vi "Three Sensors.vi"() -> ()   [LabVIEW 2019]
uses:
  <vilib>/Platform/TimedLoop/XDataNode/timing_clust.ctl
  <vilib>/Platform/TimedLoop/XDataNode/nitl_modes.ctl
  <vilib>/Platform/TimedLoop/XDataNode/wakeup.ctl
  <vilib>/myRIO/Instrument Drivers/Onboard IO/I2C/typedefs/I2C User Configuration.ctl
  <vilib>/myRIO/Instrument Drivers/Onboard IO/I2C/typedefs/I2C Transfer Rate.ctl
  <vilib>/myRIO/Instrument Drivers/Onboard IO/I2C/typedefs/I2C Reference.ctl
  <vilib>/myRIO/Common/Instrument Driver Framework/Utilities/typedefs/myRIO Generic Hardware Reference.ctl
  <vilib>/myRIO/Common/Instrument Driver Framework/Utilities/typedefs/Hardware Version Enum.ctl
  <vilib>/myRIO/Common/Instrument Driver Framework/Utilities/typedefs/myRIO v1.0 Reference.ctl
  <vilib>/myRIO/Common/Instrument Driver Framework/Utilities/typedefs/Generic FPGA Reference.ctl
  <vilib>/myRIO/Common/Instrument Driver Framework/myRIO v1.0/I2C/typedefs/I2C Channels Enum.ctl
  <vilib>/myRIO/Instrument Drivers/Onboard IO/I2C/typedefs/I2C Configuration.ctl
  <vilib>/userDefined/High Color/nirio_resource_hc.ctl
  <vilib>/myRIO/Common/Instrument Driver Framework/Utilities/vis/Is FPGA Ref Available.vi
  <vilib>/myRIO/Common/Instrument Driver Framework/myRIO v1.0/I2C/vis/myRIO v1.1 Open I2C.vi
  <vilib>/myRIO/Instrument Drivers/Onboard IO/I2C/vis/Configure.vi
  <vilib>/myRIO/Instrument Drivers/Onboard IO/I2C/vis/Write.vi
  <vilib>/myRIO/Instrument Drivers/Onboard IO/I2C/vis/Write Read.vi
  <vilib>/myRIO/Common/Instrument Driver Framework/Utilities/vis/Validate Channels.vi
  <vilib>/myRIO/Common/Instrument Driver Framework/myRIO v1.0/I2C/vis/myRIO v1.0 Reserve I2C.vi
  <vilib>/myRIO/Common/Instrument Driver Framework/myRIO v1.0/UART/vis/myRIO v1.0 Close UART.vi
  <vilib>/myRIO/Common/Instrument Driver Framework/myRIO v1.0/I2C/vis/myRIO v1.0 Build MUX Configuration I2C.vi
  <vilib>/myRIO/Common/Instrument Driver Framework/myRIO v1.0/Resource Manager/vis/myRIO v1.0 Reserve Channel List.vi
  <vilib>/myRIO/Common/Instrument Driver Framework/myRIO v1.0/Resource Manager/vis/myRIO v1.0 Create Configuration List.vi
  <vilib>/myRIO/Common/Instrument Driver Framework/myRIO v1.0/Resource Manager/vis/myRIO v1.0 Reserve Channel.vi
  <vilib>/myRIO/Common/Instrument Driver Framework/myRIO v1.0/Resource Manager/vis/myRIO v1.0 Unreserve Channel.vi
  <vilib>/myRIO/Common/Instrument Driver Framework/myRIO v1.0/Resource Manager/vis/myRIO v1.0 Build Mutex Name.vi
  <vilib>/Utility/VariantDataType/GetNumericInfo.vi
  <vilib>/Utility/error.llb/Error Cluster From Error Code.vi
  <vilib>/myRIO/Common/Instrument Driver Framework/myRIO v1.0/myRIO v1.1 Open.vi
  <vilib>/myRIO/Common/Instrument Driver Framework/Utilities/vis/IO Manager.vi
  <vilib>/myRIO/Common/Instrument Driver Framework/Utilities/vis/Configuration Manager.vi
  <vilib>/myRIO/Common/Instrument Driver Framework/myRIO v1.0/Resource Manager/vis/myRIO v1.0 Configure IO.vi
  <vilib>/myRIO/Common/Instrument Driver Framework/myRIO v1.0/myRIO v1.0 Close.vi
  <vilib>/myRIO/Common/Instrument Driver Framework/myRIO v1.0/I2C/vis/myRIO v1.0 Configure I2C.vi
  <vilib>/myRIO/Common/Instrument Driver Framework/myRIO v1.0/I2C/vis/myRIO v1.0 Write I2C.vi
  <vilib>/myRIO/Common/Instrument Driver Framework/myRIO v1.0/I2C/vis/myRIO v1.0 Read I2C.vi
  <vilib>/myRIO/Common/Instrument Driver Framework/Utilities/vis/FPGA Ref Manager.vi
  <vilib>/myRIO/Common/Instrument Driver Framework/myRIO v1.0/myRIO v1.0 Reset FPGA.vi
  <vilib>/myRIO/Common/Instrument Driver Framework/myRIO v1.0/IRQ/vis/myRIO v1.0 IRQ Info FGV.vi
  <vilib>/myRIO/Common/Instrument Driver Framework/myRIO v1.0/IRQ/vis/myRIO v1.0 Timer IRQ Info FGV.vi
  <vilib>/myRIO/Common/Instrument Driver Framework/myRIO v1.0/IRQ/vis/myRIO v1.0 ISR Agent.vi
  <vilib>/myRIO/Instrument Drivers/Utilities/vis/Reset Index.vi
  <vilib>/myRIO/Common/Instrument Driver Framework/myRIO v1.0/Resource Manager/vis/myRIO v1.0 Block Write Resource Manager.vi
  <vilib>/platform/TimedLoop/XDataNode/XDataNode.xnode
  <vilib>/myRIO/Express VI/Onboard IO/I2C/I2C Express VI.xnode
  <vilib>/myRIO/Instrument Drivers/Onboard IO/I2C/vis/myRIO I2C Open.xnode
  <vilib>/myRIO/Instrument Drivers/Utilities/Utilities.lvlib
  <vilib>/Platform/TimedLoop/XDataNode/XDNodeRunTimeDep.lvlib
  <vilib>/myRIO/Instrument Drivers/Onboard IO/I2C/I2C.lvlib
panel:
  out "Magnetic field [G] 72-1":cluster{dbl, dbl, dbl}(graph) caption="Waveform Chart"
  out "Magnetic field [G] 74-2":cluster{dbl, dbl, dbl}(graph) caption="Waveform Chart"
  out "Magnetic field [G] 74-1":cluster{dbl, dbl, dbl}(graph) caption="Waveform Chart"
  out "Z_mag 6":dbl
  out "Y_mag 6":dbl
  out "X_mag 6":dbl
  out "Z 6":i16
  out "Y 6":i16
  out "X 6":i16
  out "DATA1 6":u8[](array[numeric]) format="%02x"
  out "Z_mag 5":dbl
  out "Y_mag 5":dbl
  out "X_mag 5":dbl
  out "Z 5":i16
  out "Y 5":i16
  out "X 5":i16
  out "DATA1 5":u8[](array[numeric]) format="%02x"
  out "Z_mag 4":dbl
  out "Y_mag 4":dbl
  out "X_mag 4":dbl
  out "Z 4":i16
  out "Y 4":i16
  out "X 4":i16
  out "DATA1 4":u8[](array[numeric]) format="%02x"
  out "appended array":u8[](array[numeric])
  in  "[ESC]":bool
  # "Magnetic Sensing"
  # "DATA_X_H"
  # "DATA_X_L"
  # "DATA_Z_H"
  # "DATA_Z_L"
  # "DATA_Y_H"
  # "DATA_Y_L"
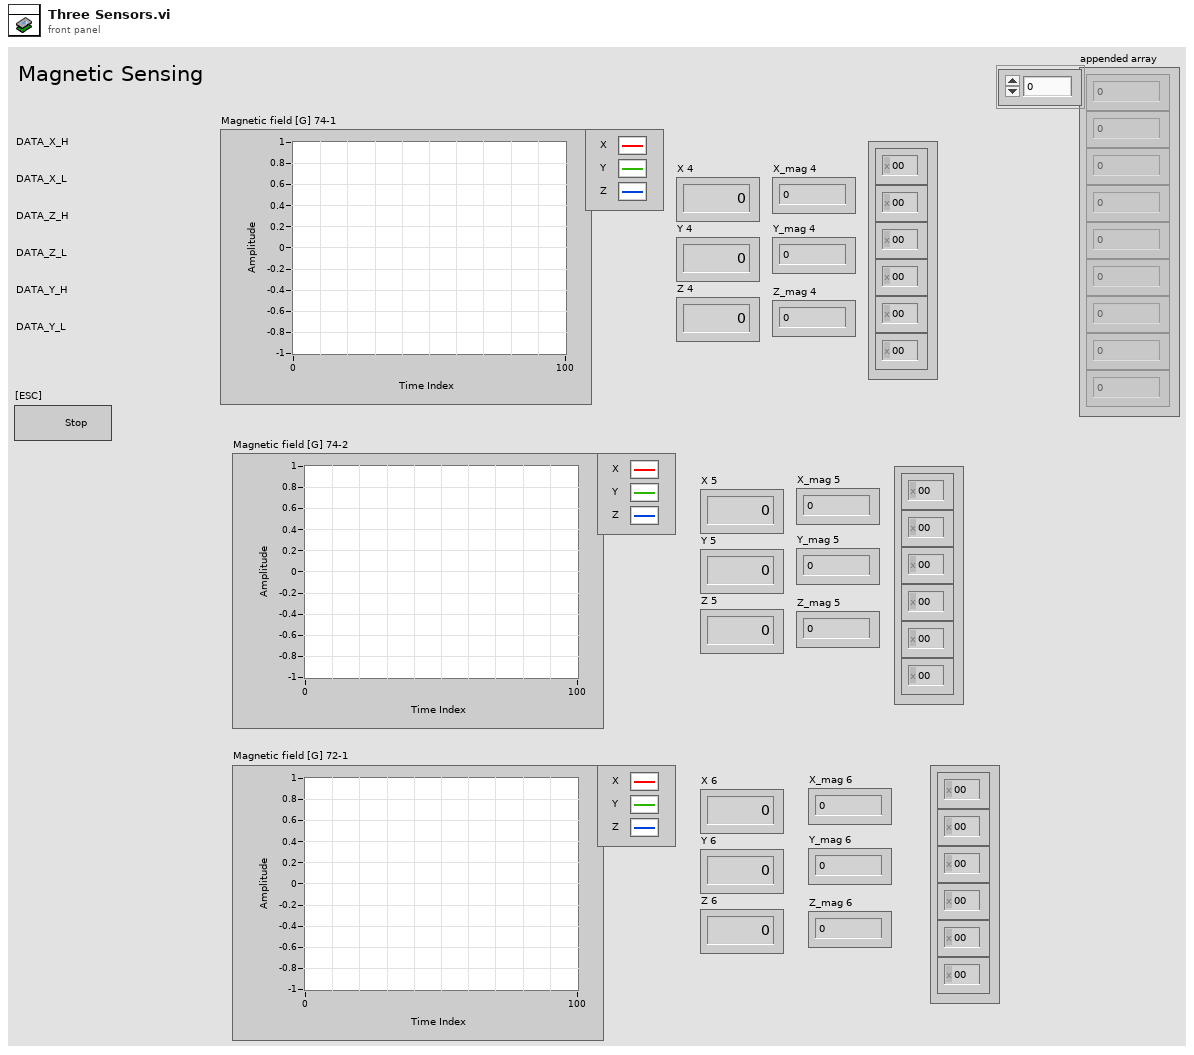
[diagram p1: front panel]
types:
  T1 = typedef "XDNodeRunTimeDep.lvlib/timing_clust.ctl" = cluster{"Expected End [f-1]":u64, "Actual End [f-1]":u64, "Finished Late? [f-1]":bool, "Expected End [i-1]":u64, "Actual End [i-1]":u64, "Finished Late? [i-1]":bool, "Expected Start [i]":u64, "Actual Start [i]":u64, "Expected Start [f]":u64, "Actual Start [f]":u64, "Source Name":string, "Structure Name":string, "Period":i64, "Deadline":i64, "Offset":i64, "Start":i64, "Priority":i32, "Timeout":i32, "Mode":T2, "Wakeup Reason":T3, "Error":errorcluster, "Source Type":string, "Secondary Source Type":string, "Global End Time":u64, "Global Start Time":u64, "Frame Duration":u64, "Iteration Duration":u64, "Assigned CPU":i32, "I/O Scan Engine Mode":u32}
  T2 = typedef "XDNodeRunTimeDep.lvlib/nitl_modes.ctl" = enum32{"No Change", "Process missed periods, maintain original phase", "Discard missed periods, maintain original phase", "Process missed periods, ignore original phase", "Discard missed periods, ignore original phase"}
  T3 = typedef "XDNodeRunTimeDep.lvlib/wakeup.ctl" = enum32{"Normal", "Aborted", "Asynchronous wakeup", "Timing source error", "Timed loop error", "Timeout"}
  T4 = typedef "I2C.lvlib/I2C Reference.ctl" = cluster{"myRIO Reference":T5, "I2C Channels Enum":T9, "I2C Configuration":T10}
  T5 = typedef "myRIO Generic Hardware Reference.ctl" = cluster{"myRIO Model":T6, "myRIO Hardware Reference":T7}
  T6 = typedef "Hardware Version Enum.ctl" = enum16{"Unknown", "myRIO-1900", "myRIO-1950", "roboRIO", "NI ELVIS RIO CM", "ELVIS III"}
  T7 = typedef "myRIO v1.0 Reference.ctl" = cluster{"Generic FPGA Reference":T8, "Allow multiple opens":bool}
  T8 = typedef "Generic FPGA Reference.ctl" = refnum<k20>
  T9 = typedef "I2C Channels Enum.ctl" = enum16{"Not Connected", "A/I2C", "B/I2C", "I2C/I2C"}
  T10 = typedef "I2C.lvlib/I2C Configuration.ctl" = cluster{"I2C Transfer Rate":T11}
  T11 = typedef "I2C.lvlib/I2C Transfer Rate.ctl" = enum16{"Standard mode (100 kbps)", "Fast mode (400 kbps)"}
  T12 = typedef "I2C.lvlib/I2C User Configuration.ctl" = cluster{"I2C Transfer Rate":T11}
  T13 = typedef "nirio_resource_hc.ctl" = tag
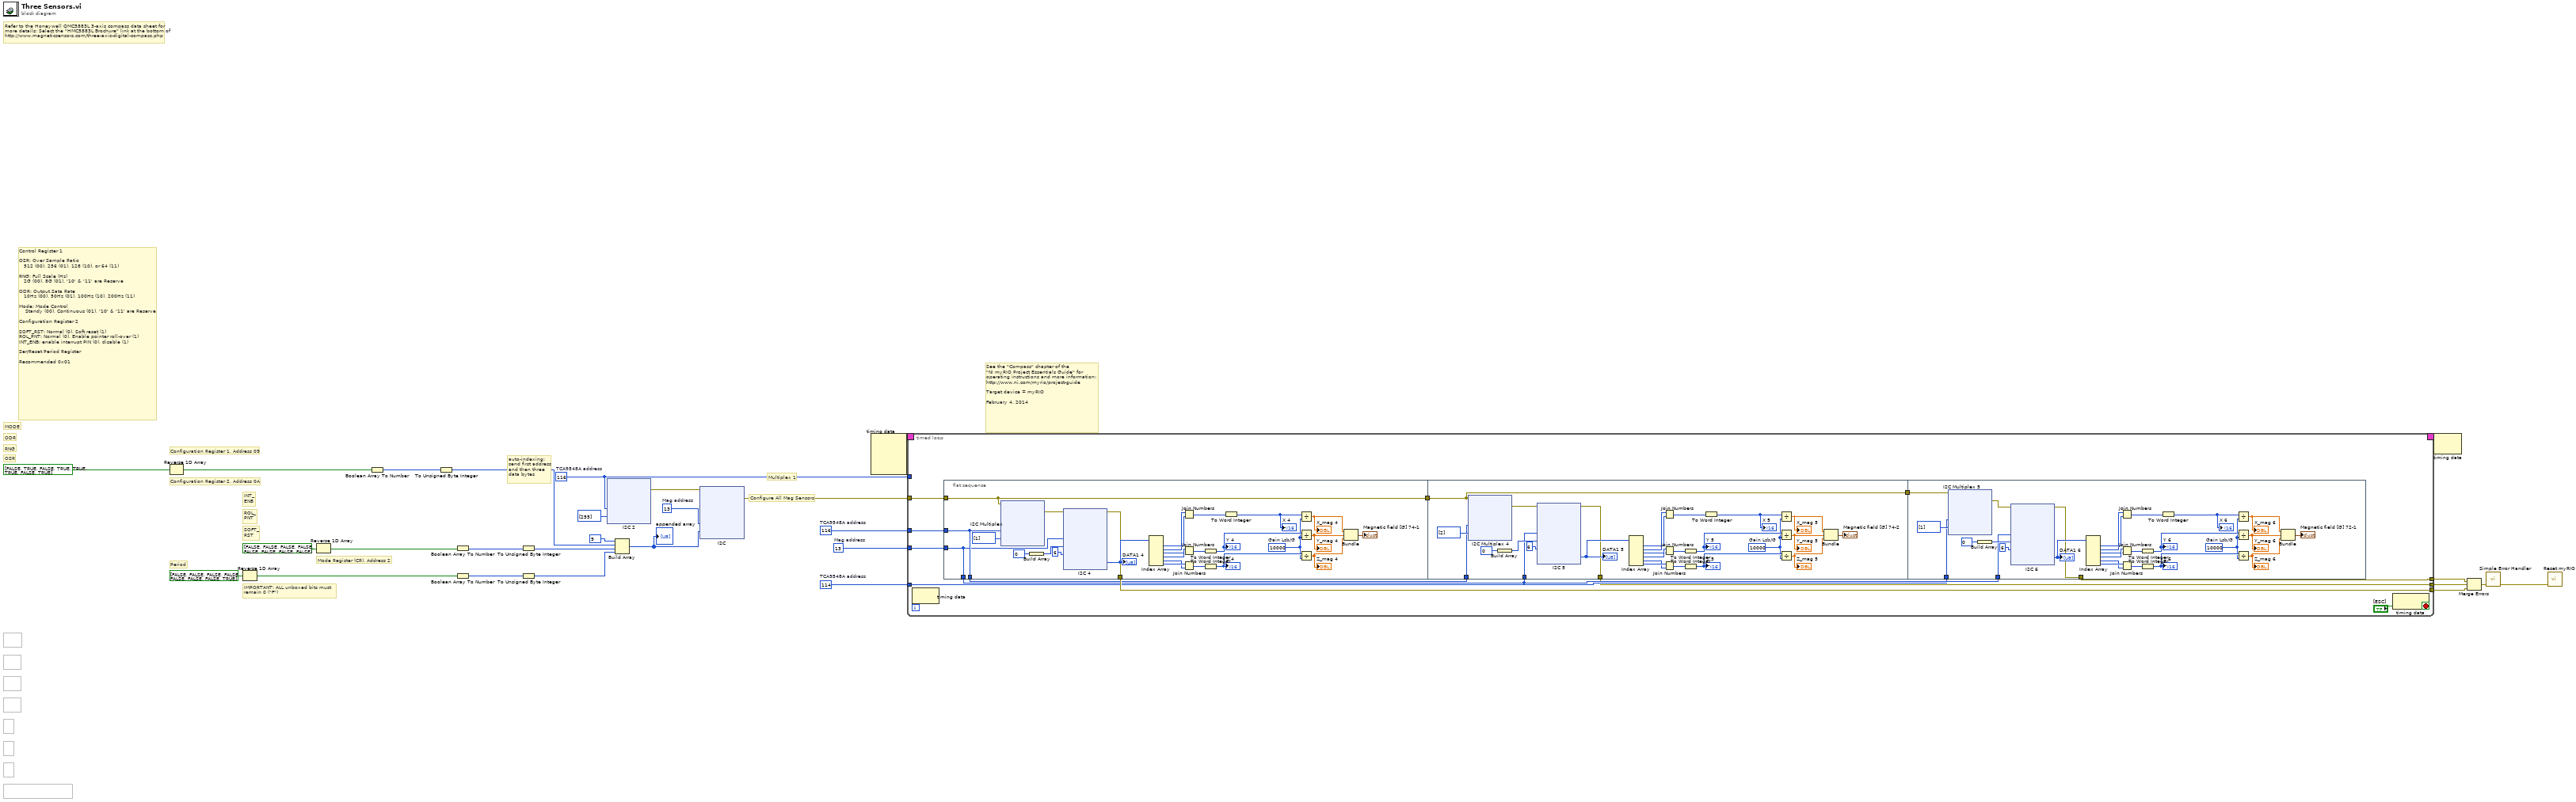
[diagram p0: block diagram]
diagram:
  w1 = u8 114  # TCA9548A address
  w2 = u8 13  # Mag address
  w3 = u8 116  # TCA9548A address
  w9 = u8 116  # TCA9548A address
  w4 = u8 13  # Mag address
  # "Multiplex 1"
  # "INT_\nENB"
  # "ROL_\nPNT"
  # "ODR"
  # "See the \"Compass\" chapter of the\n\"NI myRIO Project Essentials Guide\" for\noperating instructions and more information: \nhttp://www.ni.com/myrio/project-guide\n\nTarget device = myRIO\n\nFebruary 4, 2014"
  # "Refer to the Honeywell QMC5883L 3-axis compass data sheet for \nmore details: Select the \"HMC5883L Brochure\" link at the bottom of\nhttp://www.magneticsensors.com/three-axis-digital-compass.php"
  # "auto-indexing:\nsend first address\nand then three\ndata bytes"
  # "Control Register 1\n\nOSR: Over Sample Ratio \n   512 (00), 256 (01), 128 (10), or 64 (11)\n\nRNG: Full Scale (Hz)\n   2G (00), 8G (01), '10' & '11' are Reserve\n\nODR: Output Sata Rate\n   10Hz (00), 50Hz (01), 100Hz (10), 200Hz (11)\n\nMode: Mode Control\n    Standy (00), Continuous (01), '10' & '11' are Reserve     \n\nConfiguration Register 2\n\nSOFT_RST: Normal (0), Soft reset (1)\nROL_PNT: Normal (0), Enable pointer roll-over (1)\nINT_ENB: enable interrupt PIN (0), disable (1)\n\nSer/Reset Period Register\n\nRecommended 0x01"
  # "IMPORTANT: ALL unboxed bits must\nremain 0 (\"F\")"
  # "Configure All Mag Sensors"
  # "Period"
  # "Mode Register (CR), Address 2"
  # "Configuration Register 2, Address 0A"
  # "SOFT_\nRST"
  # "Configuration Register 1, Address 09"
  # "MODE"
  # "RNG"
  # "OSR"
  n1 = Reverse 1D Array(array=bool[] [FALSE, TRUE, FALSE, TRUE, TRUE, TRUE, FALSE, TRUE]) -> (reversed array=w25:bool[])
  n2 = Reverse 1D Array(array=bool[] [FALSE, FALSE, FALSE, FALSE, FALSE, FALSE, FALSE, TRUE]) -> (reversed array=w22:bool[])
  n3 = Reverse 1D Array(array=bool[] [FALSE, FALSE, FALSE, FALSE, FALSE, FALSE, FALSE, FALSE]) -> (reversed array=w24:bool[])
  n4 = Boolean Array To Number(Boolean array=w25) -> (number=w19:u32)
  n5 = To Unsigned Byte Integer(number=w19) -> (unsigned 8bit integer=w16:u8)
  n6 = Boolean Array To Number(Boolean array=w24) -> (number=w18:u32)
  n7 = Boolean Array To Number(Boolean array=w22) -> (number=w17:u32)
  n8 = To Unsigned Byte Integer(number=w18) -> (unsigned 8bit integer=w14:u8)
  n9 = To Unsigned Byte Integer(number=w17) -> (unsigned 8bit integer=w13:u8)
  n10 = xnode "I2C 2"("Slave Address (7-bit)"=w9, "Bytes to Write"=u8[] [255]) -> ("error out"=w11:errorcluster)  [unwired: 1 in]
  n11 = Build Array "Build Array"(u8 9 ("address"), w16, w14, w13) -> (w15:u8[])
  "appended array" <- w15
  n12 = xnode "I2C"("Slave Address (7-bit)"=w4, "Bytes to Write"=w15, "error in (no error)"=w11) -> ("error out"=w10:errorcluster)
  n13 = node-c288() -> (w28:T1)  [unwired: 4 in]
  n14 = timed-loop {
    tunnel: [w30] -> w8
    timing: w28 -> [_]
    timing-out: [_] -> w27
    tunnel: w10 -> [w39]
    tunnel: w9 -> [_]
    tunnel: [w31] -> w7
    tunnel: [w40] -> w6
    tunnel: w3 -> [w36]
    tunnel: w2 -> [w34]
    tunnel: w1 -> [w32]
    stop <- "[ESC]" stop-if-true
    n15 = node-c288() -> ()  [unwired: 1 in, 1 out]
    n16 = flat-sequence {
      tunnel: [w46] -> w40
      tunnel: w39 -> [w44]
      tunnel: [w44] -> w38
      tunnel: w36 -> [w43]
      tunnel: [w43] -> w35
      tunnel: w34 -> [w42]
      tunnel: [w42] -> w33
      tunnel: [w150] -> w31
      tunnel: w38 -> [w149]
      tunnel: [w149] -> w37
      tunnel: w35 -> [w148]
      tunnel: w33 -> [w147]
      tunnel: w37 -> [w255]
      tunnel: w33 -> [w254]
      tunnel: w32 -> [w253]
      tunnel: [w252] -> _
      tunnel: [w252] -> w30
      frame #0 {
        w58 = i16 10000  # Gain Lsb/G
        n17 = xnode "I2C Multiplex"("Slave Address (7-bit)"=w43, "Bytes to Write"=u8[] [1], "error in (no error)"=w44) -> ("error out"=w67:errorcluster)
        n18 = Build Array(u8 0) -> (w45:u8[])
        n19 = xnode "I2C 4"("Slave Address (7-bit)"=w42, "Bytes to Write"=w45, "Byte Count"=u32 6, "error in (no error)"=w67) -> ("Bytes Read"=w48:u8[], "error out"=w46:errorcluster)
        "DATA1 4" <- w48
        n20 = Index Array "Index Array"(array=w48) -> (element #1=w54:u8, element #2=w53:u8, element #3=w51:u8, element #4=w52:u8, element #5=w49:u8, element #6=w50:u8)  [unwired: 6 in]
        n21 = Join Numbers(hi=w53, lo=w54) -> ((hi.lo)=w64:u16)
        n22 = Join Numbers(hi=w52, lo=w51) -> ((hi.lo)=w62:u16)
        n23 = Join Numbers(hi=w50, lo=w49) -> ((hi.lo)=w63:u16)
        n24 = To Word Integer(number=w62) -> (16bit integer=w60:i16)
        "Y 4" <- w60
        n25 = To Word Integer(number=w63) -> (16bit integer=w59:i16)
        "Z 4" <- w59
        n26 = To Word Integer(number=w64) -> (16bit integer=w61:i16)
        "X 4" <- w61
        n27 = Divide(x=w61, y=w58) -> (x/y=w57:dbl)
        "X_mag 4" <- w57
        n28 = Divide(x=w60, y=w58) -> (x/y=w56:dbl)
        "Y_mag 4" <- w56
        n29 = Divide(x=w59, y=w58) -> (x/y=w55:dbl)
        "Z_mag 4" <- w55
        n30 = Bundle(w57, w56, w55) -> (→"Magnetic field [G] 74-1":cluster{dbl, dbl, dbl})  [unwired: 1 in]
      }
      frame #1 {
        w163 = i16 10000  # Gain Lsb/G
        n31 = xnode "I2C Multiplex 4"("Slave Address (7-bit)"=w148, "Bytes to Write"=u8[] [2], "error in (no error)"=w149) -> ("error out"=w173:errorcluster)
        n32 = Build Array(u8 0) -> (w171:u8[])
        n33 = xnode "I2C 5"("Slave Address (7-bit)"=w147, "Bytes to Write"=w171, "Byte Count"=u32 6, "error in (no error)"=w173) -> ("Bytes Read"=w153:u8[], "error out"=w150:errorcluster)
        "DATA1 5" <- w153
        n34 = Index Array "Index Array"(array=w153) -> (element #1=w159:u8, element #2=w158:u8, element #3=w156:u8, element #4=w157:u8, element #5=w154:u8, element #6=w155:u8)  [unwired: 6 in]
        n35 = Join Numbers(hi=w158, lo=w159) -> ((hi.lo)=w169:u16)
        n36 = Join Numbers(hi=w157, lo=w156) -> ((hi.lo)=w167:u16)
        n37 = Join Numbers(hi=w155, lo=w154) -> ((hi.lo)=w168:u16)
        n38 = To Word Integer(number=w167) -> (16bit integer=w165:i16)
        "Y 5" <- w165
        n39 = To Word Integer(number=w168) -> (16bit integer=w164:i16)
        "Z 5" <- w164
        n40 = To Word Integer(number=w169) -> (16bit integer=w166:i16)
        "X 5" <- w166
        n41 = Divide(x=w166, y=w163) -> (x/y=w162:dbl)
        "X_mag 5" <- w162
        n42 = Divide(x=w165, y=w163) -> (x/y=w161:dbl)
        "Y_mag 5" <- w161
        n43 = Divide(x=w164, y=w163) -> (x/y=w160:dbl)
        "Z_mag 5" <- w160
        n44 = Bundle(w162, w161, w160) -> (→"Magnetic field [G] 74-2":cluster{dbl, dbl, dbl})  [unwired: 1 in]
      }
      frame #2 {
        w267 = i16 10000  # Gain Lsb/G
        n45 = xnode "I2C Multiplex 5"("Slave Address (7-bit)"=w253, "Bytes to Write"=u8[] [1], "error in (no error)"=w255) -> ("error out"=w277:errorcluster)
        n46 = Build Array(u8 0) -> (w275:u8[])
        n47 = xnode "I2C 6"("Slave Address (7-bit)"=w254, "Bytes to Write"=w275, "Byte Count"=u32 6, "error in (no error)"=w277) -> ("Bytes Read"=w257:u8[], "error out"=w252:errorcluster)
        "DATA1 6" <- w257
        n48 = Index Array "Index Array"(array=w257) -> (element #1=w263:u8, element #2=w262:u8, element #3=w260:u8, element #4=w261:u8, element #5=w258:u8, element #6=w259:u8)  [unwired: 6 in]
        n49 = Join Numbers(hi=w262, lo=w263) -> ((hi.lo)=w273:u16)
        n50 = Join Numbers(hi=w261, lo=w260) -> ((hi.lo)=w271:u16)
        n51 = Join Numbers(hi=w259, lo=w258) -> ((hi.lo)=w272:u16)
        n52 = To Word Integer(number=w271) -> (16bit integer=w269:i16)
        "Y 6" <- w269
        n53 = To Word Integer(number=w272) -> (16bit integer=w268:i16)
        "Z 6" <- w268
        n54 = To Word Integer(number=w273) -> (16bit integer=w270:i16)
        "X 6" <- w270
        n55 = Divide(x=w270, y=w267) -> (x/y=w266:dbl)
        "X_mag 6" <- w266
        n56 = Divide(x=w269, y=w267) -> (x/y=w265:dbl)
        "Y_mag 6" <- w265
        n57 = Divide(x=w268, y=w267) -> (x/y=w264:dbl)
        "Z_mag 6" <- w264
        n58 = Bundle(w266, w265, w264) -> (→"Magnetic field [G] 72-1":cluster{dbl, dbl, dbl})  [unwired: 1 in]
      }
    }
    n59 = node-c288() -> ()  [unwired: 1 in, 1 out]
  }
  n60 = node-c288(w27) -> ()  [unwired: 1 out]
  n61 = Merge Errors(w8, w7, w6) -> (w5:errorcluster)
  n62 = call <vilib>:"Simple Error Handler.vi"("error in (no error)"=w5) -> ("error out"=w29:errorcluster)  [unwired: 4 in, 4 out]
  n63 = call <vilib>:"Reset myRIO.vi"("error in (no error)"=w29) -> ()  [unwired: 10 in, 1 out]
